vi "BCM_CmdStr_287.vi"(1 "BCM命令输入":T1 {"实际天窗位置" items=["位置未知", "完全关闭", "完全打开", "倾斜与张开之间", "完全倾斜", "倾斜与关闭之间", "滑动开启舒适位置", "预留"]; "天窗水平开度值" min=0 max=100 step=1 scale=0.0..100.0; "天窗运行状态" items=["Not Pressed", "Manual slide open", "Manual slide close", "Manual tilt open", "Manual tilt close", "Auto slide open", "Auto slide close", "Auto tilt open", "Auto tilt close", "Moving uninitialized", "Reversing", "Reserved"]}) -> (0 "CmdStr":string)   [LabVIEW 2013]
uses:
  BCM_287.ctl
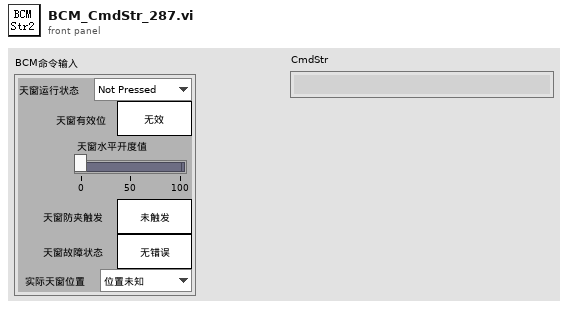
[diagram p1: front panel]
types:
  T1 = typedef "BCM_287.ctl" = cluster{"天窗运行状态":u16, "天窗有效位":bool, "天窗水平开度值":i32, "天窗防夹触发":bool, "天窗故障状态":bool, "实际天窗位置":u16}
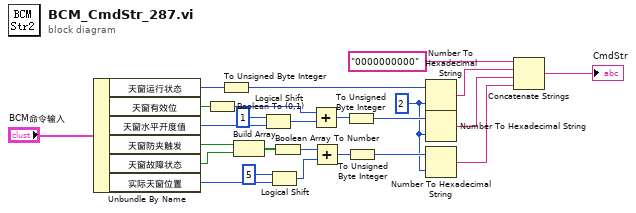
[diagram p0: block diagram]
diagram:
  w2 = 2
  n1 = Unbundle By Name("BCM命令输入") -> ("天窗运行状态"=w24:u16, "天窗有效位"=w23:bool, "天窗水平开度值"=w22:i32, "天窗防夹触发"=w17:bool, "天窗故障状态"=w16:bool, "实际天窗位置"=w13:u16)
  n2 = Boolean To (0,1)(Boolean=w23) -> (0, 1=w19:i16)
  n3 = To Unsigned Byte Integer(number=w24) -> (unsigned 8bit integer=w8:u8)
  n4 = Build Array(w17, w16) -> (w15:bool[])
  n5 = Logical Shift(y=u8 1, x=w22) -> (x << y=w20:i32)
  n6 = Logical Shift(y=u8 5, x=w13) -> (x << y=w11:u16)
  n7 = Boolean Array To Number(Boolean array=w15) -> (number=w12:u32)
  n8 = Add(x=w19, y=w20) -> (x+y=w18:i32)
  n9 = Add(x=w12, y=w11) -> (x+y=w10:u32)
  n10 = To Unsigned Byte Integer(number=w18) -> (unsigned 8bit integer=w7:u8)
  n11 = To Unsigned Byte Integer(number=w10) -> (unsigned 8bit integer=w6:u8)
  n12 = Number To Hexadecimal String(1:w2, 2:w8) -> (0:w5:string)
  n13 = Number To Hexadecimal String(1:w2, 2:w7) -> (0:w4:string)
  n14 = Number To Hexadecimal String(1:w2, 2:w6) -> (0:w3:string)
  n15 = Concatenate Strings("0000000000", w5, w4, w3) -> (→"CmdStr":string)
